vi "FPGA TEST.vi"() -> ()   [LabVIEW 2017]
uses:
  <vilib>/rvi/Emulation/niFpgaGetClockAttributes.vi
  <vilib>/rvi/Emulation/niFpgaSctlEmulationGetInTimedLoop.vi
  <vilib>/rvi/Emulation/niFpgaEmulationReportErrorSimple.vi
  <vilib>/rvi/eio/common/nirviEmuTemplateMethod_errors.vi
  <vilib>/rvi/Emulation/niFpgaCriticalErrorInLSC.vi
  <vilib>/eio/EIONode/EIONode.xnode
  <vilib>/eio/EIOMethodNode/EIOMethodNode.xnode
panel:
  out "pulse width (uSec)":u32
  out "timed out?":bool
  out "ENC 5":i32
  in  "Reset ENC 5":bool
  out "ENC 3":i32
  in  "Reset ENC 3":bool
  out "ENC 2":i32
  in  "Reset ENC 2":bool
  out "ENC 4":i32
  in  "Reset ENC 4":bool
  out "ENC 1":i32
  in  "Reset ENC 1":bool
  out "ENC 6":i32
  in  "Reset ENC 6":bool
  in  "A/DIO6":bool
  in  "B/DIO7":bool
  in  "A/DIO4":bool
  in  "A/DIO13":bool
  in  "A/DIO5":bool
  in  "A/DIO7":bool
  in  "T 4":u32
  in  "F 4":u32
  in  "T 3":u32
  in  "F 3":u32
  in  "T 2":u32
  in  "F 2":u32
  in  "T":u32
  in  "F":u32
  # "PWM"
  # "DIR"
  # "ENC"
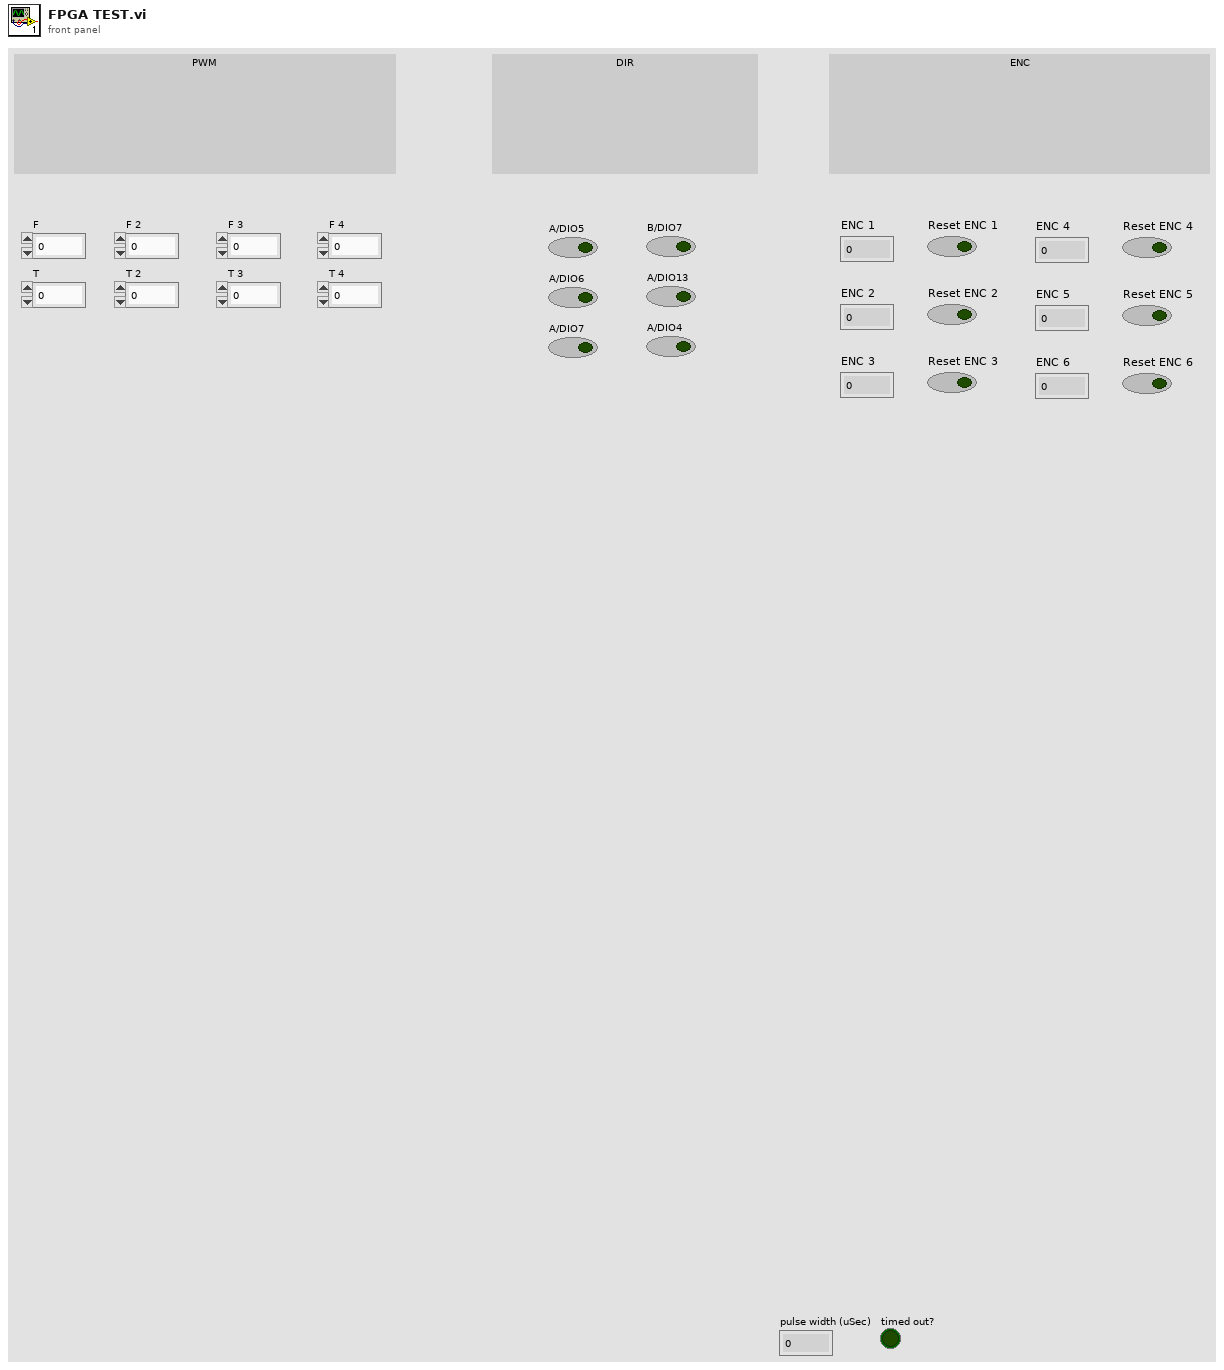
[diagram p1: front panel]
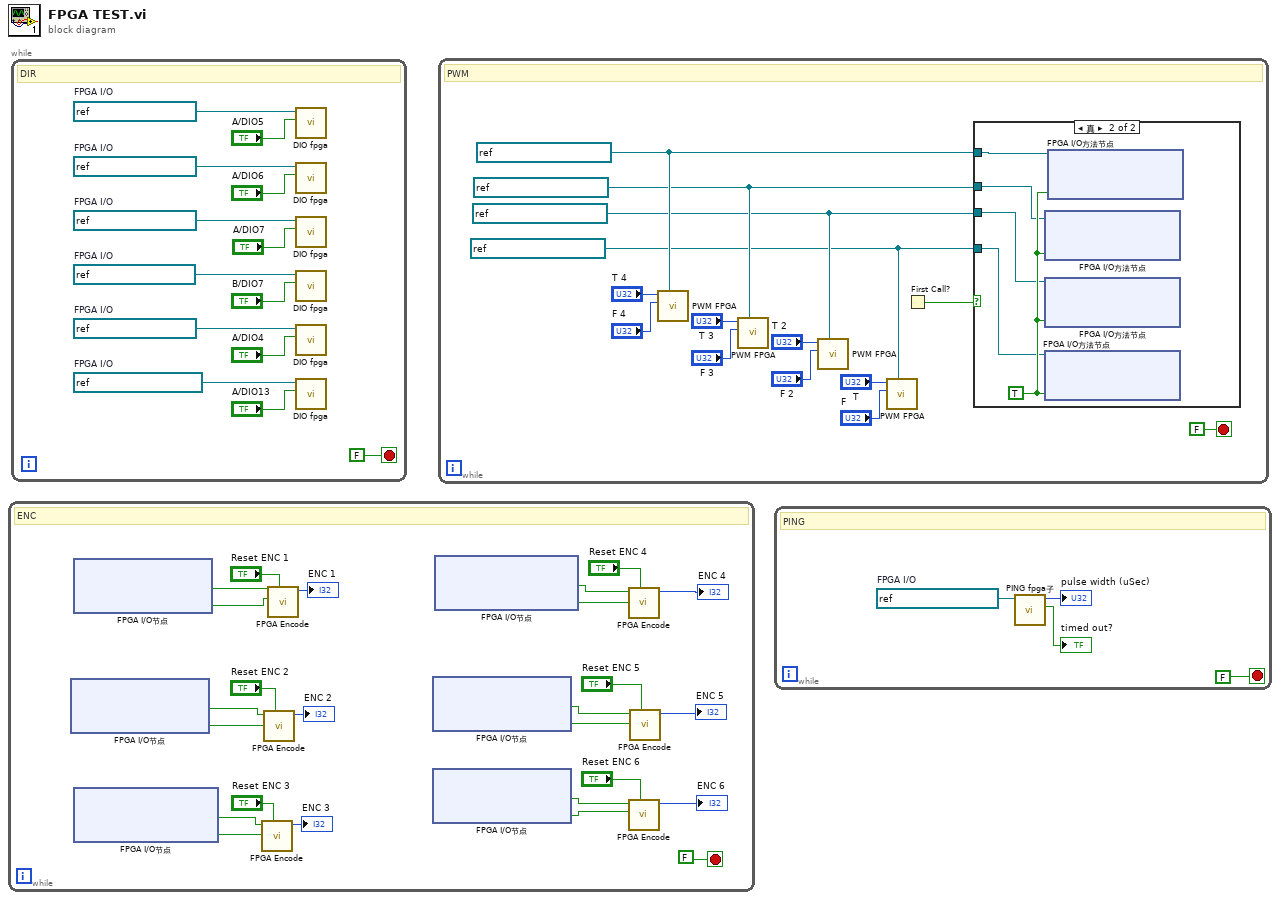
[diagram p0: block diagram]
diagram:
  n1 = while {
    stop <- FALSE ("停止") stop-if-true
    # "ENC"
    n2 = xnode "FPGA I/O节点"() -> ("ConnectorA/DIO2"=w22:bool, "ConnectorA/DIO3"=w21:bool)  [unwired: 2 in, 2 out]
    n3 = xnode "FPGA I/O节点"() -> ("ConnectorA/DIO0"=w24:bool, "ConnectorA/DIO1"=w23:bool)  [unwired: 2 in, 2 out]
    n4 = xnode "FPGA I/O节点"() -> ("ConnectorA/DIO11"=w20:bool, "ConnectorA/DIO12"=w19:bool)  [unwired: 2 in, 2 out]
    n5 = call "FPGA Encode.vi"("Reset ENC1"="Reset ENC 3", "B"=w19, "A"=w20) -> ("ENC"=→"ENC 3":i32)  [unwired: 8 in]
    n6 = call "FPGA Encode.vi"("Reset ENC1"="Reset ENC 2", "B"=w21, "A"=w22) -> ("ENC"=→"ENC 2":i32)  [unwired: 8 in]
    n7 = call "FPGA Encode.vi"("Reset ENC1"="Reset ENC 1", "B"=w23, "A"=w24) -> ("ENC"=→"ENC 1":i32)  [unwired: 8 in]
    n8 = xnode "FPGA I/O节点"() -> ("ConnectorC/DIO0"=w16:bool, "ConnectorC/DIO2"=w15:bool)  [unwired: 2 in, 2 out]
    n9 = xnode "FPGA I/O节点"() -> ("ConnectorC/DIO4"=w14:bool, "ConnectorC/DIO6"=w13:bool)  [unwired: 2 in, 2 out]
    n10 = xnode "FPGA I/O节点"() -> ("ConnectorB/DIO11"=w18:bool, "ConnectorB/DIO12"=w17:bool)  [unwired: 2 in, 2 out]
    n11 = call "FPGA Encode.vi"("Reset ENC1"="Reset ENC 4", "B"=w17, "A"=w18) -> ("ENC"=→"ENC 4":i32)  [unwired: 8 in]
    n12 = call "FPGA Encode.vi"("Reset ENC1"="Reset ENC 6", "B"=w13, "A"=w14) -> ("ENC"=→"ENC 6":i32)  [unwired: 8 in]
    n13 = call "FPGA Encode.vi"("Reset ENC1"="Reset ENC 5", "B"=w15, "A"=w16) -> ("ENC"=→"ENC 5":i32)  [unwired: 8 in]
  }
  n14 = while {
    stop <- FALSE stop-if-true
    w33 = refnum<k21> "ConnectorA/DIO13"  # FPGA I/O
    w34 = refnum<k21> "ConnectorA/DIO4"  # FPGA I/O
    w35 = refnum<k21> "ConnectorB/DIO7"  # FPGA I/O
    w36 = refnum<k21> "ConnectorA/DIO7"  # FPGA I/O
    w37 = refnum<k21> "ConnectorA/DIO6"  # FPGA I/O
    w38 = refnum<k21> "ConnectorA/DIO5"  # FPGA I/O
    # "DIR"
    n15 = call "DIO fpga.vi"("I/O项"="A/DIO5", "引用句柄输入"=w38) -> ()  [unwired: 10 in]
    n16 = call "DIO fpga.vi"("I/O项"="A/DIO6", "引用句柄输入"=w37) -> ()  [unwired: 10 in]
    n17 = call "DIO fpga.vi"("I/O项"="A/DIO7", "引用句柄输入"=w36) -> ()  [unwired: 10 in]
    n18 = call "DIO fpga.vi"("I/O项"="B/DIO7", "引用句柄输入"=w35) -> ()  [unwired: 10 in]
    n19 = call "DIO fpga.vi"("I/O项"="A/DIO4", "引用句柄输入"=w34) -> ()  [unwired: 10 in]
    n20 = call "DIO fpga.vi"("I/O项"="A/DIO13", "引用句柄输入"=w33) -> ()  [unwired: 10 in]
  }
  n21 = while {
    stop <- FALSE stop-if-true
    w47 = refnum<k21> "ConnectorA/DIO8" ("FPGA I/O In")
    w48 = refnum<k21> "ConnectorA/DIO9" ("FPGA I/O In")
    w49 = refnum<k21> "ConnectorA/DIO10" ("FPGA I/O In")
    w50 = refnum<k21> "ConnectorB/DIO8" ("FPGA I/O In")
    # "PWM"
    n22 = call "PWM FPGA.vi"("引用句柄输入"=w50, "F"="F 4", "T"="T 4") -> ()  [unwired: 9 in]
    n23 = call "PWM FPGA.vi"("引用句柄输入"=w49, "F"="F 3", "T"="T 3") -> ()  [unwired: 9 in]
    n24 = call "PWM FPGA.vi"("引用句柄输入"=w48, "F"="F 2", "T"="T 2") -> ()  [unwired: 9 in]
    n25 = call "PWM FPGA.vi"("引用句柄输入"=w47, "F"="F", "T"="T") -> ()  [unwired: 9 in]
    n26 = First Call?() -> (First Call?: T/F=w51:bool)
    n27 = case shown="真" w51 {
      tunnel: w50 -> [_ w57]
      tunnel: w49 -> [_ w55]
      tunnel: w48 -> [_ w54]
      tunnel: w47 -> [_ w53]
      frame False {
      }
      frame True {
        w56 = TRUE ("Enable")
        n28 = xnode "FPGA I/O方法节点"("FPGA I/O In"=w55, "Enable"=w56) -> ()  [unwired: 1 out]
        n29 = xnode "FPGA I/O方法节点"("FPGA I/O In"=w54, "Enable"=w56) -> ()  [unwired: 1 out]
        n30 = xnode "FPGA I/O方法节点"("FPGA I/O In"=w53, "Enable"=w56) -> ()  [unwired: 1 out]
        n31 = xnode "FPGA I/O方法节点"("FPGA I/O In"=w57, "Enable"=w56) -> ()  [unwired: 1 out]
      }
    }
  }
  n32 = while {
    stop <- FALSE stop-if-true
    w58 = refnum<k21> "ConnectorB/DIO1"  # FPGA I/O
    # "PING"
    n33 = call "PING fpga子.vi"("引用句柄输入"=w58) -> ("timed out?"=→"timed out?":bool, "pulse width (uSec)"=→"pulse width (uSec)":u32)  [unwired: 9 in]
  }
